vi "VI Tree - lvdata__ogtk.vi"() -> ()   [LabVIEW 2019]
uses:
  Type Descriptor Enumeration__ogtk.ctl
  Type Descriptor Header__ogtk.ctl
  Refnum Code__ogtk.ctl
  Base Units__ogtk.ctl
  Physical Units__ogtk.ctl
  Type Descriptor__ogtk.ctl
  Waveform Subtype Enum__ogtk.ctl
  Refnum Subtype Enum__ogtk.ctl
panel:
  in  "Refnum Subtype Enum":T1 format="%.0x"
  in  "Waveform Subtype Enum":T2 format="%.0x"
  in  "Type Descriptor":T3
  in  "Physical Units":T4
  in  "Base Units":T5
  in  "Refnum Code":T6
  out "Type Descriptor Header":T7 {"type" format="%.0x"}
  in  "Type Descriptor Enumeration":T8 format="%.0x"
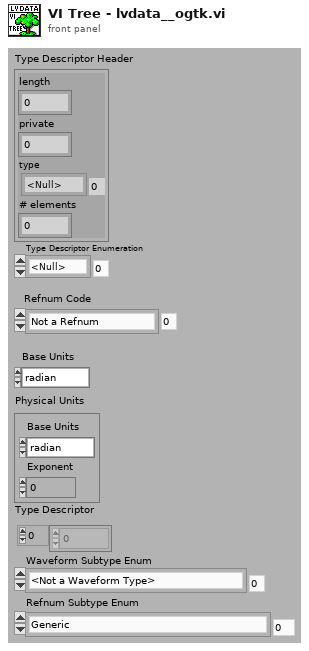
[diagram p1: front panel]
types:
  T1 = typedef "Refnum Subtype Enum__ogtk.ctl" = enum8{"Generic", "Datalog File Refnum", "Byte Stream File Refnum", "Device Refnum", "Occurence Refnum", "TCP Connection Refnum", "VISA Refnum (Obsolete)", "Automation Renum", "VI Server Refnum", "Menu Refnum", "IVI Refnum (Obsolete)", "IMAQ Session", "0x0C", "Datasocket Refnum", "VISA Resource", "IVI Logical Name", "UDP Connection Refnum", "Notifier Refnum", "Queue Refnum", "IrDA Refnum", "Hardware Plugin Refnum", "Hardware Plugin Tag Refnum", "DAQmx Refnum", "Event Registration Refnum", ".NET Refnum", "User Event Refnum", "0x1A", "Event Callback", "0x1C", "0x1D", "LabVIEW Class Instance", "Bluetooth", "Data Value References", "RT FIFO", "TDM Streaming"}
  T2 = typedef "Waveform Subtype Enum__ogtk.ctl" = enum8{"<Not a Waveform Type>", "0x01", "Analog 16-bit signed", "Analog Double-Precision", "0x04", "Analog Single Precision", "Timestamp", "Digital Data", "Digital Waveform", "Dynamic Data", "Analog Extended-Precision", "Analog 8-bit unsigned", "Analog 16-bit unsigned", "Analog 32-bit unsigned", "Analog 8-bit signed", "Analog 32-bit signed", "Analog Complex Single-Precision", "Analog Complex Double-Precision", "Analog Complex Extended Precision", "Analog 64-bit signed", "Analog 64-bit unsigned"}
  T3 = typedef "Type Descriptor__ogtk.ctl" = i16[]
  T4 = typedef "Physical Units__ogtk.ctl" = cluster{"Base Units":enum16{"radian", "steradian", "second", "meter", "kilogram", "ampere", "kelvin", "mole", "candela"}, "Exponent":i16}
  T5 = typedef "Base Units__ogtk.ctl" = enum16{"radian", "steradian", "second", "meter", "kilogram", "ampere", "kelvin", "mole", "candela"}
  T6 = typedef "Refnum Code__ogtk.ctl" = enum16{"Not a Refnum", "Datalog File", "Byte Stream File", "0x03", "Occurence", "TCP", "0x06", "ActiveX", "Generic VI Server Class", "Menu", "0x0A", "IMAQ Session", "0x0C", "0x0D", "VISA", "IVI", "UDP"}
  T7 = typedef "Type Descriptor Header__ogtk.ctl" = cluster{"length":u16, "private":u8, "type":T8, "# elements":u16}
  T8 = typedef "Type Descriptor Enumeration__ogtk.ctl" = enum8{"<Null>", "I8", "I16", "I32", "I64", "U8", "U16", "U32", "U64", "SGL", "DBL", "EXT", "CSG", "CDB", "CXT", "0x0F", "0x10", "0x11", "0x12", "0x13", "0x14", "Enum U8", "Enum U16", "Enum U32", "Enum U64", "SGL PQ", "DBL PQ", "EXT PQ", "CSG PQ", "CDB PQ", "CXT PQ", "0x1F", "0x20", "Boolean", "0x22", "0x23", "0x24", "0x25", "0x26", "0x27", "0x28", "0x29", "0x2A", "0x2B", "0x2C", "0x2D", "0x2E", "0x2F", "String", "0x31", "Path", "Pict", "0x34", "0x35", "0x36", "DAQ", "0x38", "0x39", "0x3A", "0x3B", "0x3C", "0x3D", "0x3E", "0x3F", "Array", "0x41", "0x42", "0x43", "0x44", "0x45", "0x46", "0x47", "0x48", "0x49", "0x4A", "0x4B", "0x4C", "0x4D", "0x4E", "0x4F", "Cluster", "0x51", "0x52", "Variant", "Waveform", "0x55", "0x56", "0x57", "0x58", "0x59", "0x5A", "0x5B", "0x5C", "0x5D", "0x5E", "Fixed Point", "0x60", "0x61", "0x62", "0x63", "0x64", "0x65", "0x66", "0x67", "0x68", "0x69", "0x6A", "0x6B", "0x6C", "0x6D", "0x6E", "0x6F", "Refnum", "0x71", "0x72", "Set Collection", "Map Collection"}
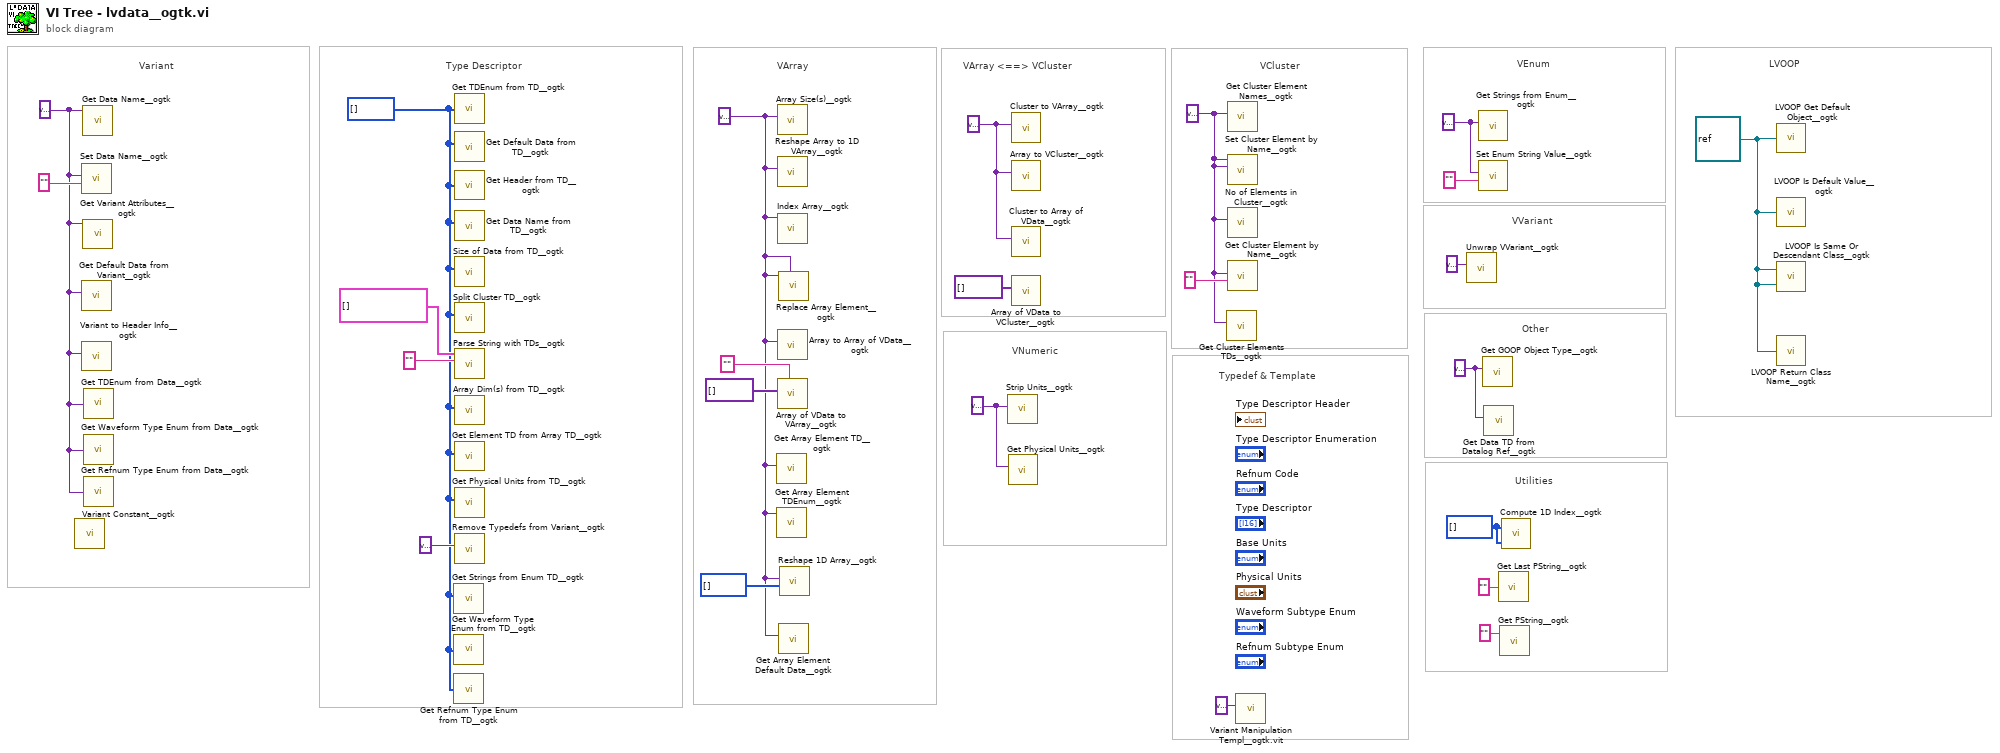
[diagram p0: block diagram]
diagram:
  w1 = refnum<class> refnum ("Object")
  w7 = variant ("Number or 1D array with units")
  w3 = variant ("Enum")
  w6 = variant ("Cluster")
  w5 = variant ("Cluster")
  w22 = u32[] [] ("Indices")
  w10 = T3 [] ("Type Descriptor")
  w4 = variant ("GOOP Refnum")
  w8 = variant ("Array")
  w2 = variant ("Data")
  # "LVOOP"
  # "VVariant"
  # "VNumeric"
  # "Other"
  # "Type Descriptor"
  # "Typedef & Template"
  # "Variant"
  # "Utilities"
  # "VEnum"
  # "VArray <==> VCluster"
  # "VCluster"
  # "VArray"
  n1 = call "Variant Constant__ogtk.vi"() -> ()  [unwired: 1 in]
  n2 = call "Set Data Name__ogtk.vi"("Data Name"="", "Data"=w2) -> ()  [unwired: 8 in, 2 out]
  n3 = call "Get Default Data from Variant__ogtk.vi"("Variant"=w2) -> ()  [unwired: 9 in, 2 out]
  n4 = call "Variant to Header Info__ogtk.vi"("Variant"=w2) -> ()  [unwired: 3 in, 3 out]
  n5 = call "Get Data Name__ogtk.vi"("Data"=w2) -> ()  [unwired: 8 in, 3 out]
  n6 = call "Get Variant Attributes__ogtk.vi"("Variant"=w2) -> ()  [unwired: 3 in, 4 out]
  n7 = call "Get TDEnum from Data__ogtk.vi"("Data"=w2) -> ()  [unwired: 4 in, 1 out]
  n8 = call "Get Waveform Type Enum from Data__ogtk.vi"("Data"=w2) -> ()  [unwired: 4 in, 1 out]
  n9 = call "Get Refnum Type Enum from Data__ogtk.vi"("Data"=w2) -> ()  [unwired: 4 in, 1 out]
  n10 = call "Get Strings from Enum TD__ogtk.vi"("Type Descriptor"=w10) -> ()  [unwired: 8 in, 3 out]
  n11 = call "Get Waveform Type Enum from TD__ogtk.vi"("Type Descriptor"=w10) -> ()  [unwired: 4 in, 1 out]
  n12 = call "Get Refnum Type Enum from TD__ogtk.vi"("Type Descriptor"=w10) -> ()  [unwired: 4 in, 1 out]
  n13 = call "Get TDEnum from TD__ogtk.vi"("Type Descriptor"=w10) -> ()  [unwired: 4 in, 1 out]
  n14 = call "Get Default Data from TD__ogtk.vi"("Type Descriptor"=w10) -> ()  [unwired: 9 in, 2 out]
  n15 = call "Get Header from TD__ogtk.vi"("Type Descriptor"=w10) -> ()  [unwired: 1 out]
  n16 = call "Get Data Name from TD__ogtk.vi"("Type Descriptor"=w10) -> ()  [unwired: 9 in, 2 out]
  n17 = call "Size of Data from TD__ogtk.vi"("Type Descriptor"=w10) -> ()  [unwired: 9 in, 2 out]
  n18 = call "Split Cluster TD__ogtk.vi"("Type Descriptor"=w10) -> ()  [unwired: 9 in, 2 out]
  n19 = call "Parse String with TDs__ogtk.vi"("Data string"="", "Type Descriptors"=cluster{"Type Descriptor":T3}[] []) -> ()  [unwired: 7 in, 3 out]
  n20 = call "Array Dim(s) from TD__ogtk.vi"("Array Type Descriptor"=w10) -> ()  [unwired: 9 in, 2 out]
  n21 = call "Get Element TD from Array TD__ogtk.vi"("Array Type Descriptor"=w10) -> ()  [unwired: 9 in, 2 out]
  n22 = call "Get Physical Units from TD__ogtk.vi"("Float or Array Type Descriptor"=w10) -> ()  [unwired: 9 in, 2 out]
  n23 = call "Remove Typedefs from Variant__ogtk.vi"("Variant with typedefs"=variant) -> ()  [unwired: 9 in, 2 out]
  n24 = call "Get Array Element TD__ogtk.vi"("Array"=w8) -> ()  [unwired: 9 in, 2 out]
  n25 = call "Get Array Element TDEnum__ogtk.vi"("Array"=w8) -> ()  [unwired: 9 in, 2 out]
  n26 = call "Array Size(s)__ogtk.vi"("Array"=w8) -> ()  [unwired: 8 in, 3 out]
  n27 = call "Reshape Array to 1D VArray__ogtk.vi"("MultiD Array"=w8) -> ()  [unwired: 8 in, 3 out]
  n28 = call "Index Array__ogtk.vi"("MultiD Array"=w8) -> ()  [unwired: 9 in, 2 out]
  n29 = call "Array to Array of VData__ogtk.vi"("MultiD Array"=w8) -> ()  [unwired: 9 in, 2 out]
  n30 = call "Array of VData to VArray__ogtk.vi"("Array Name"="", "1D Array of VData"=variant[] []) -> ()  [unwired: 8 in, 2 out]
  n31 = call "Replace Array Element__ogtk.vi"("New Element"=w8, "MultiD Array"=w8) -> ()  [unwired: 8 in, 2 out]
  n32 = call "Get Array Element Default Data__ogtk.vi"("Array"=w8) -> ()  [unwired: 9 in, 2 out]
  n33 = call "Reshape 1D Array__ogtk.vi"("Size(s)"=u32[] [], "1D Array"=w8) -> ()  [unwired: 8 in, 2 out]
  n34 = call "Strip Units__ogtk.vi"("Number or 1D array with units"=w7) -> ()  [unwired: 9 in, 2 out]
  n35 = call "Get Physical Units__ogtk.vi"("Float or Array of Floats"=w7) -> ()  [unwired: 9 in, 2 out]
  n36 = call "Cluster to VArray__ogtk.vi"("Cluster"=w6) -> ()  [unwired: 9 in, 2 out]
  n37 = call "Array to VCluster__ogtk.vi"("Array"=w6) -> ()  [unwired: 9 in, 2 out]
  n38 = call "Cluster to Array of VData__ogtk.vi"("Cluster"=w6) -> ()  [unwired: 9 in, 2 out]
  n39 = call "Array of VData to VCluster__ogtk.vi"("Array"=variant[] []) -> ()  [unwired: 9 in, 2 out]
  n40 = call "Get Cluster Elements TDs__ogtk.vi"("Cluster"=w5) -> ()  [unwired: 9 in, 2 out]
  n41 = call "Get Cluster Element Names__ogtk.vi"("Cluster"=w5) -> ()  [unwired: 9 in, 2 out]
  n42 = call "Set Cluster Element by Name__ogtk.vi"("New Element Value"=w5, "Cluster"=w5) -> ()  [unwired: 7 in, 3 out]
  n43 = call "No of Elements in Cluster__ogtk.vi"("Cluster"=w5) -> ()  [unwired: 9 in, 2 out]
  n44 = call "Get Cluster Element by Name__ogtk.vi"("Element Name"="", "Cluster"=w5) -> ()  [unwired: 7 in, 3 out]
  n45 = call "Variant Manipulation Templ__ogtk.vit"("Variant"=variant) -> ()  [unwired: 10 in, 1 out]
  n46 = call "Unwrap VVariant__ogtk.vi"("VVariant"=variant) -> ()  [unwired: 9 in, 2 out]
  n47 = call "Get Strings from Enum__ogtk.vi"("Enum"=w3) -> ()  [unwired: 7 in, 4 out]
  n48 = call "Set Enum String Value__ogtk.vi"("String Value"="", "Default Enum Value"=w3) -> ()  [unwired: 8 in, 2 out]
  n49 = call "Get GOOP Object Type__ogtk.vi"("GOOP Refnum"=w4) -> ()  [unwired: 9 in, 2 out]
  n50 = call "Get Data TD from Datalog Ref__ogtk.vi"("Datalog Refnum"=w4) -> ()  [unwired: 9 in, 2 out]
  n51 = call "Get Last PString__ogtk.vi"("String"="") -> ()  [unwired: 2 out]
  n52 = call "Get PString__ogtk.vi"("String"="") -> ()  [unwired: 1 in, 2 out]
  n53 = call "Compute 1D Index__ogtk.vi"("Size(s)"=w22, "Indices"=w22) -> ()  [unwired: 1 out]
  n54 = call "LVOOP Get Default Object__ogtk.vi"("Object"=w1) -> ()  [unwired: 1 out]
  n55 = call "LVOOP Is Default Value__ogtk.vi"("Object"=w1) -> ()  [unwired: 1 out]
  n56 = call "LVOOP Is Same Or Descendant Class__ogtk.vi"("Possible Descendant Object"=w1, "Object"=w1) -> ()  [unwired: 1 out]
  n57 = call "LVOOP Return Class Name__ogtk.vi"("Object"=w1) -> ()  [unwired: 3 out]
